vi "Dashboard Main.vi"() -> ()   [LabVIEW 2013]
uses:
  Program Files (x86)/National Instruments/LabVIEW 2013/examples/FRC/Vision/2014 Target Detection/TargetType.ctl
  <vilib>/event_ctls.llb/eventvkey.ctl
  <vilib>/Rock Robotics/WPI/Dashboard/WPI_DashboardLogging Global.vi
  <vilib>/Utility/config.llb/Write Key (String).vi
  <vilib>/Utility/config.llb/Write Key (I32).vi
  <vilib>/Utility/config.llb/NI_LVConfig.lvlib
panel:
  out "Image Message":string="Timeout in Camera Communications"
  in  "Rec Mode":enum32{"Stop", "Record", "Playback"}(radio)
  in  "Dashboard Tab":T1(tab)
  in  "Camera Settings":T2={"Frame Rate"=30, "Compression"=30, "Size"=1} {"Frame Rate" scale=1.0..30.0; "Size" items=["640x480", "320x240", "160x120"]}
  out "MotorSliders R":cluster{"MotorSlide1":dbl, "MotorSlide2":dbl} {"MotorSlide2" scale=-1.0..1.0 scale format="%#_2e"; "MotorSlide1" scale=-1.0..1.0 scale format="%#_2e"}
  out "MotorChart R":cluster{"Numeric":dbl, "Numeric":dbl}(graph)
  out "MotorSliders L":T3 {"MotorSlide4 2" scale=0.0..14.0 scale format="%#_2e"; "MotorSlide2" scale=-1.0..1.0 scale format="%#_2e"; "MotorSlide1" scale=-1.0..1.0 scale format="%#_2e"}
  out "MotorChart L":T4(graph)
  out "JS1 Z":dbl(slide) scale=-1.0..1.0 scale format="%#_2e"
  out "Joystick 1":cluster{"X":dbl, "Y":dbl}[](graph)
  out "JS Buttons 1":T5
  out "JS2 Z":dbl(slide) scale=-1.0..1.0 scale format="%#_2e"
  out "Joystick 2":cluster{"X":dbl, "Y":dbl}[](graph)
  out "JS Buttons 2":T5
  out "Mode":T6(ring)=enum."Auto Disabled"
  out "Camera IP":string
  in  "DB Camera Config":bool
  out "fps":dbl format="%#.1g"
  out "Mbps":dbl format="%#.1g"
  out "Mbps 2":bool
  out "LED 1":bool
  in  "Camera IP":string="10.21.38.11"
  out "Auto To Run":dbl
  in  "Manual Override":bool=TRUE
  out "Halo Sensitivity":dbl=0.75
  out "Ultrasonic":dbl
  in  "Vision Color Controls":T7={"Hue"={110.0, 142.0}, "Sat"={138.0, 255.0}, "Val"={139.0, 198.0}} {"Val" scale=0.0..255.0; "Sat" scale=0.0..255.0; "Hue" scale=0.0..255.0 scale format="%#_3g"}
  out "Distances":T9(array[cluster])
  in  "Test Slider":dbl(slide) scale=0.0..100.0 scale format="%#_3g"
  in  "On/Off":bool caption="Solenoid"
  in  "Test Name":u16(ring) items=["Select the test to run...", "Example Test", "-------------------------------", "List of tests is built in robot code.", "Replace with your own automated tests."]
  in  "Test Tree":string(tree)
  in  "Motor":cluster{"Value":dbl, "Enable":bool} {"Value" scale=-1.0..1.0 scale format="%#_3g"}
  out "Progress":T10 {"Test Progress" scale=0.0..100.0}
  in  "Rev/Fwd":cluster{"Forward":bool, "Reverse":bool}
  in  "Test Ring":u16(ring) items=["Auto", "Fixed indoor", "Fixed outdoor 1", "Fixed outdoor 2", "Fixed fluorescent 1", "Fixed fluorescent 2", "Hold current"]
  in  "Listbox":i32(listbox)
  out "Tree":string(tree)
  out "Camera Image":T11(plugin-control)
  in  "Enable Camera":bool=TRUE
  # "Left"
  # "Front"
  # "Right"
  # "Battery"
  # "Increment with Start,\nDecrement with Back"
  # "Increment with Right D-Pad,\nDecrement with Left D-Pad"
  # "This tab is a great place for autonomous settings and validation.\nCustomize by placing controls and indicators here and name to\nmatch Dashboard Variables on robot."
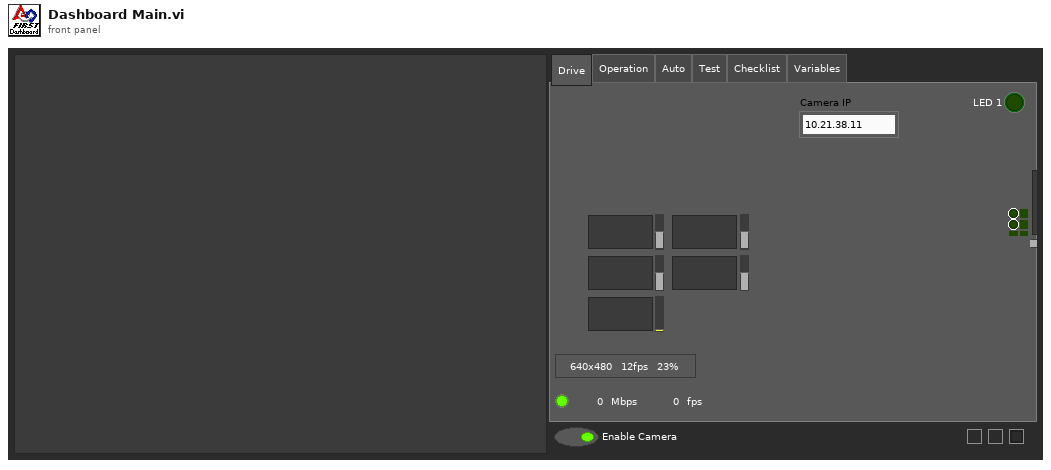
[diagram p1: front panel]
types:
  T1 = enum32{"Drive", "Operation", "Auto", "Test", "Checklist", "Variables"}
  T2 = cluster{"Frame Rate":i32, "Compression":i32, "Size":u16}
  T3 = cluster{"MotorSlide1":dbl, "MotorSlide2":dbl, "MotorSlide4 2":dbl}
  T4 = cluster{"Numeric":dbl, "Numeric":dbl, "Battery":sgl}
  T5 = cluster{bool, bool, bool, bool, bool, bool, bool, bool, bool, bool, bool, bool}
  T6 = enum8{"Tele-Op Disabled", "Tele-Op Enabled", "Auto Disabled", "Auto Enabled", "Test Disabled", "Test Enabled", ""}
  T7 = cluster{"Hue":cluster{dbl, dbl}, "Sat":cluster{dbl, dbl}, "Val":cluster{dbl, dbl}}
  T8 = typedef "TargetType.ctl" = enum16{"Not Hot", "Hot"}
  T9 = cluster{"Distance (ft)":dbl, "Target Center (-1 to 1)":cluster{"X":dbl, "Y":dbl}, "Left":bool, "State":T8}[]
  T10 = cluster{"Test Progress":u8, "Test Progress Text":string}
  T11 = typedef "IMAQ Image.ctl" = refnum<image>
  T12 = typedef "Image Type" = u32
  T13 = cluster{"Digital Inputs":bool[], "Digital Outputs":bool[]}
  T14 = cluster{"Competition mode":bool, "Robot Link":bool, "Autonomous":bool, "Enabled":bool, "E-Stop":bool, "Simulated":bool, "TestMode":bool, "Docked Window":bool}
  T15 = cluster{"Boolean Array[0]":bool, "Boolean Array[1]":bool, "Boolean Array[2]":bool, "Boolean Array[3]":bool, "Boolean Array[4]":bool, "Boolean Array[5]":bool, "Boolean Array[6]":bool, "Boolean Array[7]":bool, "Boolean Array[8]":bool, "Boolean Array[9]":bool, "Boolean Array[10]":bool, "Boolean Array[11]":bool}
  T16 = cluster{cluster{dbl, dbl}, cluster{dbl, dbl}, cluster{dbl, dbl}}
  T17 = typedef "NI_LVConfig.lvlib/Config Data RefNum.ctl" = refnum<k1>
  T18 = typedef "eventvkey.ctl" = enum16{"ASCII", "Enter", "Return", "Shift", "Ctrl", "Alt", "Cmd", "Opt", "Caps", "NumLock", "Clear", "Break", "Up", "Down", "Left", "Right", "Insert", "Delete", "Home", "End", "PageUp", "PageDown", "Escape", "Help", "Pause", "ScrollLock", "F1", "F2", "F3", "F4", "F5", "F6", "F7", "F8", "F9", "F10", "F11", "F12", "F13", "F14", "F15", "F16", "F17", "F18", "F19", "F20", "F21", "F22", "F23", "F24", "Play", "VolumeUp", "VolumeDown", "Mute", "Two Byte Char"}
  T19 = cluster{"Image Size":bool, "Image Type":bool, "Pixel Value":bool, "ROI Information":bool, "Zoom Factor":bool}
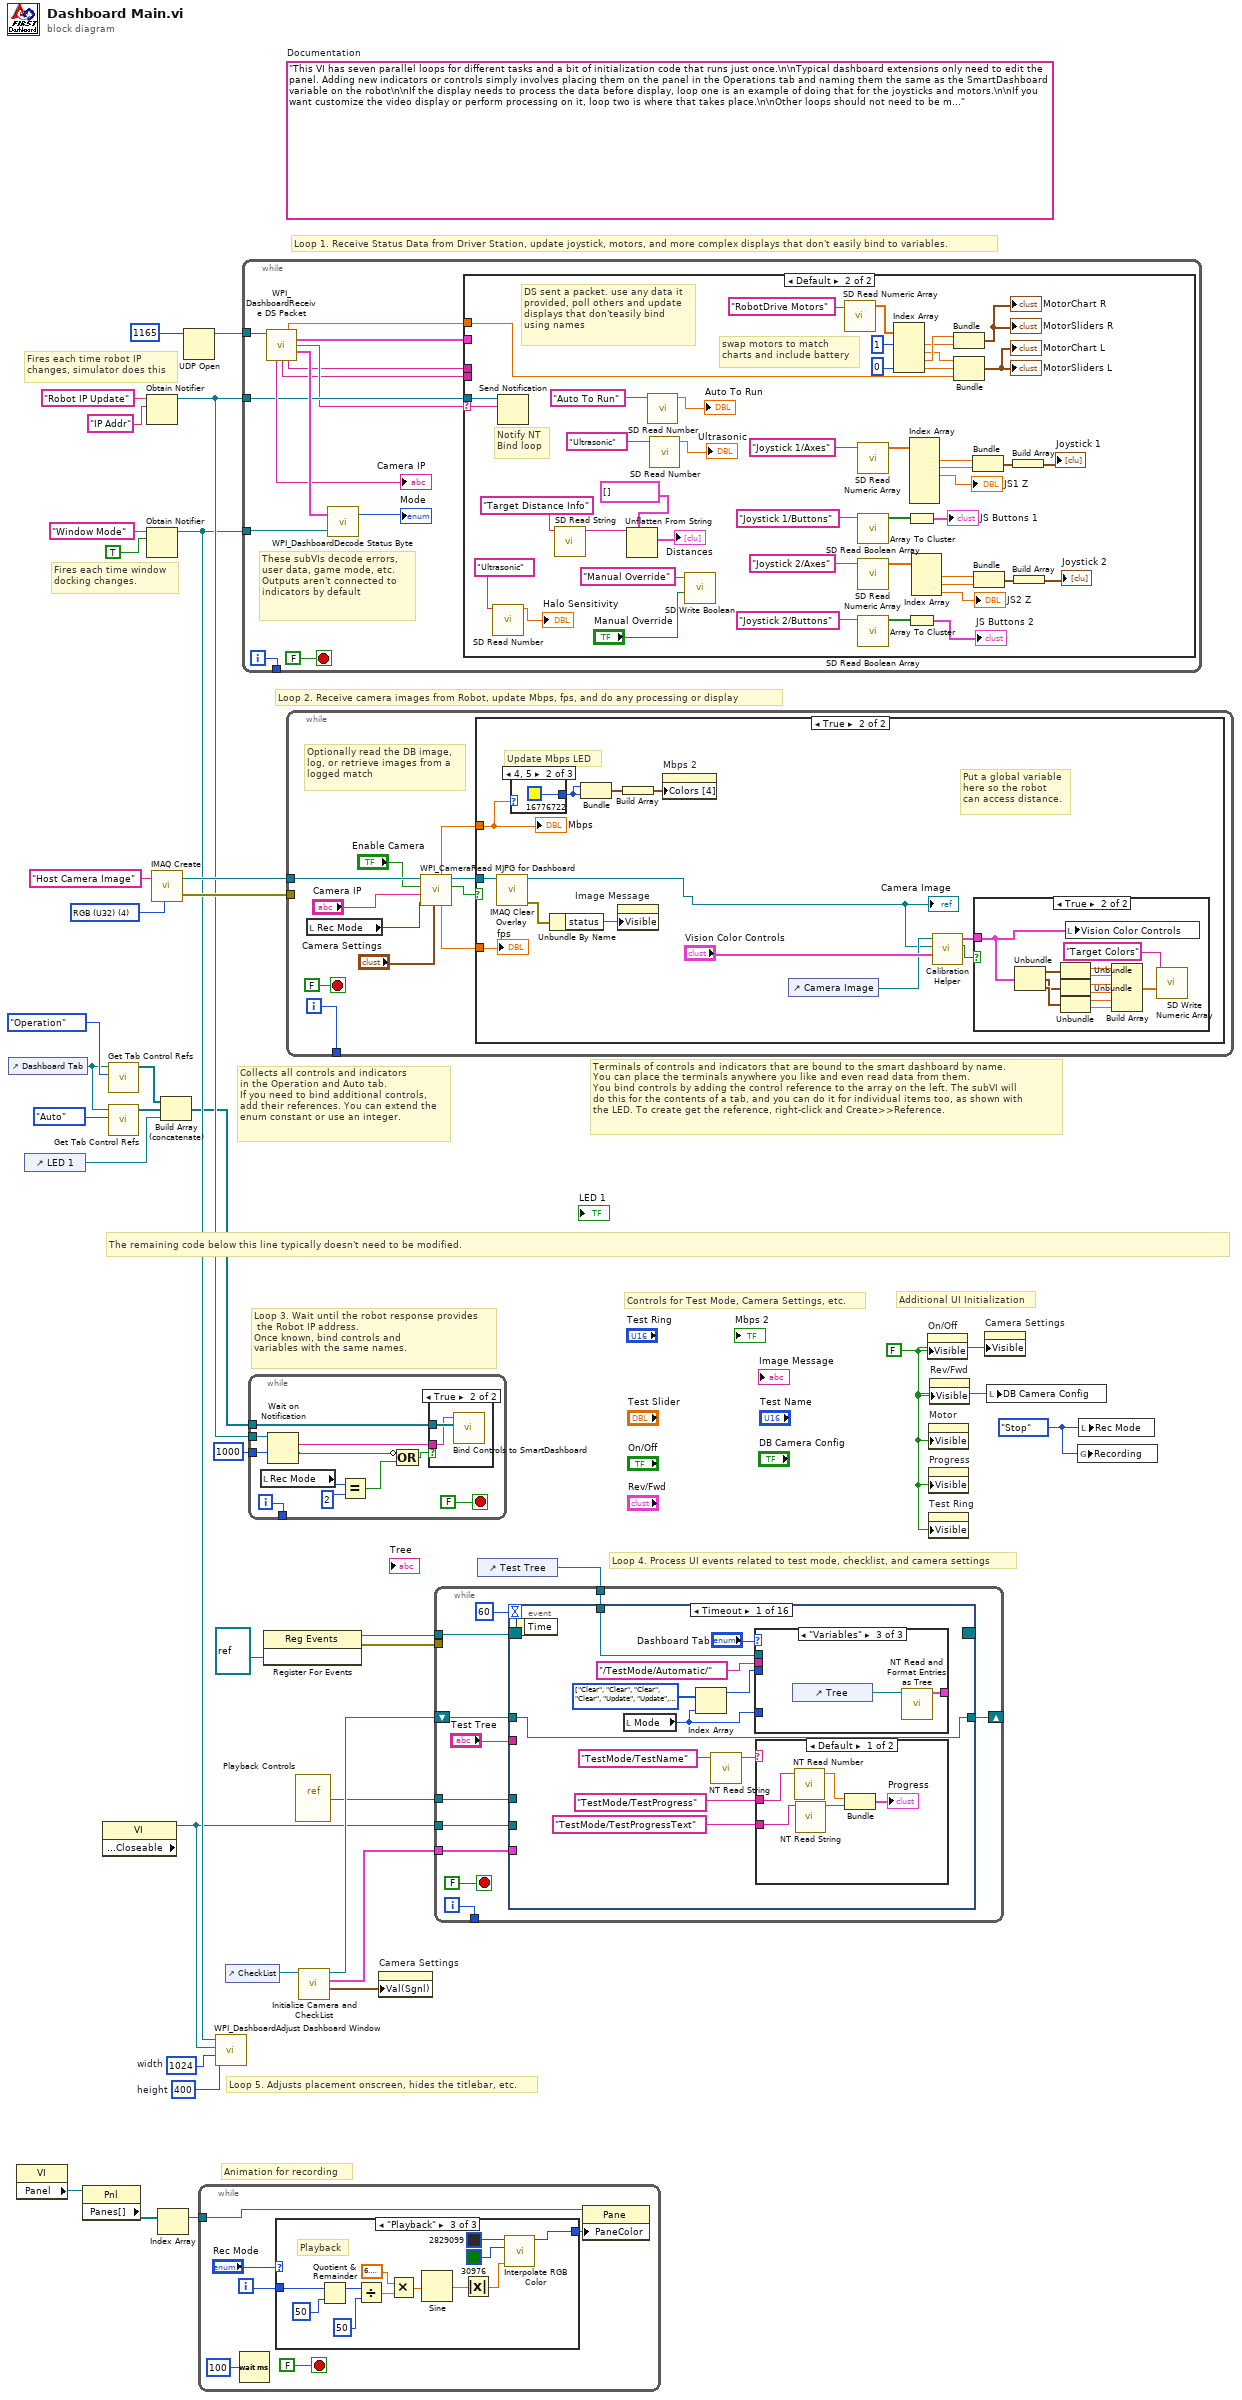
[diagram p0: block diagram]
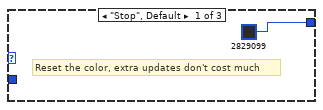
[diagram p2: hidden frame]
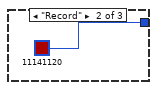
[diagram p3: hidden frame]
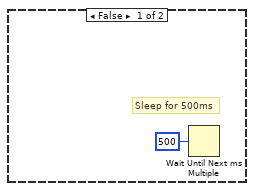
[diagram p5: hidden frame]
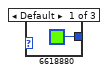
[diagram p7: hidden frame]
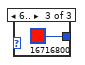
[diagram p8: hidden frame]
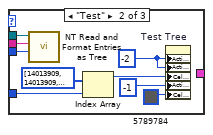
[diagram p10: hidden frame]
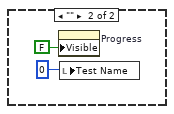
[diagram p11: hidden frame]
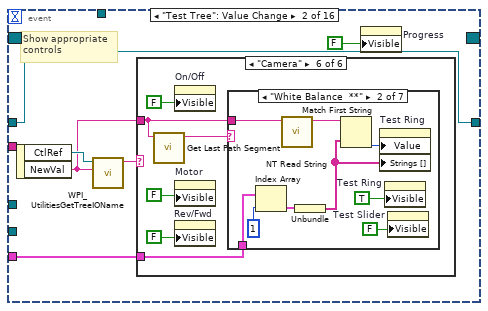
[diagram p12: hidden frame]
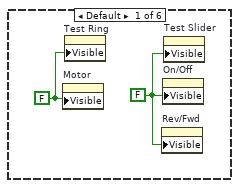
[diagram p13: hidden frame]
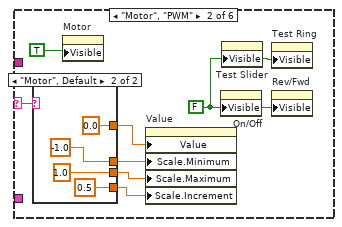
[diagram p14: hidden frame]
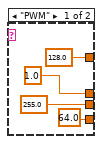
[diagram p15: hidden frame]
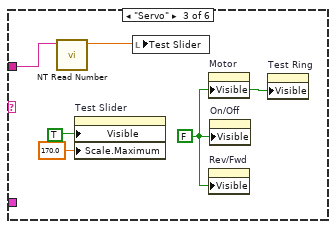
[diagram p16: hidden frame]
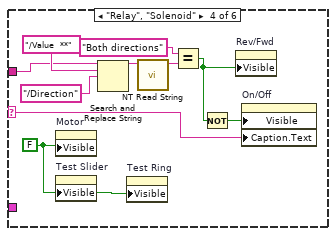
[diagram p17: hidden frame]
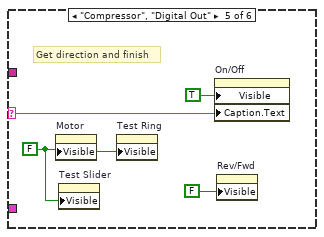
[diagram p18: hidden frame]
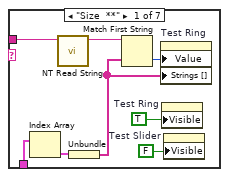
[diagram p19: hidden frame]
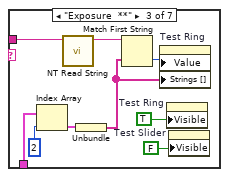
[diagram p20: hidden frame]
diagram:
  w8 = enum32{"Stop", "Record", "Playback"}."Stop" ("Rec Mode")
  w11 = 400  # height
  w12 = 1024  # width
  w25 = FALSE ("Visible")
  (unwired) "This VI has seven parallel loops for different tasks and a bit of initialization code that runs just once.\n\nTypical dashboard extensions only need to edit the panel. Adding new indicators or controls simply involves placing them on the panel in the Operations tab and naming them the same as the SmartDashboard variable on the robot\n\nIf the display needs to process the data before display, loop one is an example of doing that for the joysticks and motors.\n\nIf you want customize the video display or perform processing on it, loop two is where that takes place.\n\nOther loops should not need to be modified. They are pretty standard, and document the task they perform."  # Documentation
  w35 = T12 4 items=["Grayscale (U8)", "Grayscale (I16)", "Grayscale (SGL)", "Complex (CSG)", "RGB (U32)", "HSL (U32)", "RGB (U64)"] ("Image Type")
  # "Controls for Test Mode, Camera Settings, etc."
  # "Additional UI Initialization"
  # "Animation for recording"
  # "Fires each time robot IP\nchanges, simulator does this"
  # "Fires each time window\ndocking changes."
  # "Collects all controls and indicators\nin the Operation and Auto tab.\nIf you need to bind additional controls,\nadd their references. You can extend the\nenum constant or use an integer."
  # "The remaining code below this line typically doesn't need to be modified."
  # "Loop 4. Process UI events related to test mode, checklist, and camera settings"
  # "Terminals of controls and indicators that are bound to the smart dashboard by name.\nYou can place the terminals anywhere you like and even read data from them.\nYou bind controls by adding the control reference to the array on the left. The subVI will\ndo this for the contents of a tab, and you can do it for individual items too, as shown with\nthe LED. To create get the reference, right-click and Create>>Reference."
  # "Loop 3. Wait until the robot response provides\n the Robot IP address.\nOnce known, bind controls and\nvariables with the same names."
  # "Loop 5. Adjusts placement onscreen, hides the titlebar, etc."
  # "Loop 1. Receive Status Data from Driver Station, update joystick, motors, and more complex displays that don't easily bind to variables."
  # "Loop 2. Receive camera images from Robot, update Mbps, fps, and do any processing or display"
  n1 = control-ref of="Dashboard Tab"() -> (w6:refnum<vi>)
  n2 = property class="VI"() -> ("Panel"=w19:refnum<vi>)  [unwired: 2 in, 2 out]
  n3 = control-ref of="LED 1"() -> (w1:refnum<vi>)
  n4 = property class="Pnl"(reference=w19) -> ("Panes[]"=w20:refnum<vi>[])  [unwired: 1 in, 2 out]
  n5 = property class="VI" props=["Front Panel.Closeable"]() -> (reference out=w7:refnum<vi>)  [unwired: 2 in, 2 out]
  n6 = call <vilib>:"Get Tab Control Refs.vi"("Page Index"=T1."Operation" ("Dashboard Tab"), "TabControl in"=w6) -> ("ControlsOnPage"=w4:refnum<vi>[])  [unwired: 9 in]
  n7 = call <vilib>:"Get Tab Control Refs.vi"("Page Index"=T1."Auto" ("Dashboard Tab"), "TabControl in"=w6) -> ("ControlsOnPage"=w5:refnum<vi>[])  [unwired: 9 in]
  n8 = Obtain Notifier(name (unnamed)="Robot IP Update", notification data type="IP Addr" ("name (unnamed)")) -> (notifier out=w29:refnum<notifier>)  [unwired: 2 in, 2 out]
  n9 = Obtain Notifier(name (unnamed)="Window Mode", notification data type=TRUE) -> (notifier out=w10:refnum<notifier>)  [unwired: 2 in, 2 out]
  n10 = call "IMAQ Create"("Image Name"="Host Camera Image", "Image Type"=w35) -> ("New Image"=w33:T11, "error out"=w32:errorcluster)  [unwired: 2 in, 1 out]
  n11 = Index Array(array=w20) -> (element=w18:refnum<vi>)  [unwired: 1 in]
  n12 = Build Array (concatenate)(w4, w5, w1) -> (w3:refnum<vi>[])
  n13 = UDP Open(11:u16 1165 ("port")) -> (port=w36:refnum<k16>)  [unwired: 2 in, 4 out]
  n14 = while {
    tunnel: w18 -> [w39]
    i -> [w42]
    stop <- FALSE stop-if-true
    n15 = Wait (ms)(milliseconds to wait=u32 100) -> ()  [unwired: 1 out]
    n16 = case shown="\"Playback\"" "Rec Mode" {
      tunnel: w42 -> [_ _ w57]
      tunnel: [u32 2829099 ("Base Color") u32 11141120 ("Target Color") w46] -> w38
      frame "Stop", Default {
        # "Reset the color, extra updates don't cost much"
      }
      frame "Record" {
      }
      frame "Playback" {
        # "Playback"
        n17 = Quotient & Remainder(x=w57, y=u32 50 ("milliseconds to wait")) -> (x-y*floor(x/y)=w53:u32)  [unwired: 1 out]
        n18 = Divide(x=w53, y=u32 50 ("milliseconds to wait")) -> (x/y=w50:dbl)
        n19 = Multiply(x=6.283185307179586, y=w50) -> (x*y=w55:dbl)
        n20 = Sine(x=w55) -> (sin(x)=w54:dbl)
        n21 = Absolute Value(x=w54) -> (abs(x)=w47:dbl)
        n22 = call "Interpolate RGB Color.vi"("Proportion"=w47, "Target Color"=u32 30976, "Base Color"=u32 2829099) -> ("Result Color"=w46:u32)  [unwired: 8 in]
      }
    }
    n23 = property class="Pane"(reference=w39, "PaneColor"=w38) -> ()  [unwired: 1 in, 2 out]
  }
  n24 = call <vilib>:"WPI_DashboardAdjust Dashboard Window.vi"("height"=w11, "width"=w12, "reference in"=w7, "Notifier in"=w10) -> ()  [unwired: 8 in]
  n25 = control-ref of="CheckList"() -> (w9:refnum<vi>)
  n26 = while {
    tunnel: w36 -> [w68]
    tunnel: w29 -> [w63]
    tunnel: w10 -> [w67]
    tunnel: [w64] -> _
    i -> [w64]
    stop <- FALSE stop-if-true
    # "These subVIs decode errors, user data, game mode, etc.\nOutputs aren't connected to indicators by default"
    n27 = call <vilib>:"WPI_DashboardReceive DS Packet.vi"("Recv Socket"=w68) -> ("Battery"=w58:sgl, "Driver Station"=w59:T13, "Robot IP Address"=w62:string, "Status"=w69:T14, "Camera IP Address"=→"Camera IP":string, "Low Priority User Data"=w61:string, "High Priority User Data"=w60:string)  [unwired: 1 in, 7 out]
    n28 = call <vilib>:"WPI_DashboardDecode Status Byte.vi"("Window Mode Notifier"=w67, "Status"=w69) -> ("Mode"=→"Mode":T6)  [unwired: 1 out]
    n29 = case shown="Default" w62 {
      selector: w62 -> [_ w94]
      tunnel: w63 -> [_ w95]
      tunnel: w61 -> [_ _]
      tunnel: w60 -> [_ _]
      tunnel: w59 -> [_ _]
      tunnel: w58 -> [_ w93]
      frame "0.0.0.0" {
        # "DS not sending packets, or no robot exists yet.\nDon't poll the variables"
      }
      frame Default {
        # "Notify NT\nBind loop"
        # "DS sent a packet. use any data it\nprovided, poll others and update\ndisplays that don'teasily bind\nusing names"
        # "swap motors to match\ncharts and include battery"
        n30 = call <vilib>:"SD Read Number.vi"("Name"="Ultrasonic") -> ("Numeric"=→"Halo Sensitivity":dbl)  [unwired: 8 in, 2 out]
        n31 = Send Notification(notification=w94, notifier=w95) -> ()  [unwired: 1 in, 2 out]
        n32 = call <vilib>:"SD Read String.vi"("Name"="Target Distance Info") -> ("String"=w80:string)  [unwired: 8 in, 2 out]
        n33 = Unflatten From String(type=T9 [] ("Distances"), binary string=w80) -> (value=→"Distances":T9)  [unwired: 3 in, 2 out]
        n34 = call <vilib>:"SD Read Number.vi"("Name"="Auto To Run") -> ("Numeric"=→"Auto To Run":dbl)  [unwired: 8 in, 2 out]
        n35 = call <vilib>:"SD Read Number.vi"("Name"="Ultrasonic") -> ("Numeric"=→"Ultrasonic":dbl)  [unwired: 8 in, 2 out]
        n36 = call <vilib>:"SD Write Boolean.vi"("Boolean"="Manual Override", "Name"="Manual Override") -> ()  [unwired: 8 in, 2 out]
        n37 = call <vilib>:"SD Read Numeric Array.vi"("Name"="RobotDrive Motors") -> ("Numeric Array"=w92:dbl[])  [unwired: 8 in, 2 out]
        n38 = call <vilib>:"SD Read Numeric Array.vi"("Name"="Joystick 1/Axes") -> ("Numeric Array"=w110:dbl[])  [unwired: 8 in, 2 out]
        n39 = call <vilib>:"SD Read Boolean Array.vi"("Name"="Joystick 1/Buttons") -> ("Boolean Array"=w112:bool[])  [unwired: 8 in, 2 out]
        n40 = call <vilib>:"SD Read Numeric Array.vi"("Name"="Joystick 2/Axes") -> ("Numeric Array"=w105:dbl[])  [unwired: 8 in, 2 out]
        n41 = call <vilib>:"SD Read Boolean Array.vi"("Name"="Joystick 2/Buttons") -> ("Boolean Array"=w104:bool[])  [unwired: 8 in, 2 out]
        n42 = Index Array(array=w92, index #1=1, index #4=0) -> (element #1=w88:dbl, element #2=w87:dbl, element #3=w89:dbl, element #4=w84:dbl)  [unwired: 2 in]
        n43 = Array To Cluster(array=w112) -> (cluster=→"JS Buttons 1":T15)
        n44 = Array To Cluster(array=w104) -> (cluster=→"JS Buttons 2":T15)
        n45 = Index Array(array=w110) -> (element #1=w108:dbl, element #2=w79:dbl, element #3=→"JS1 Z":dbl)  [unwired: 6 in, 3 out]
        n46 = Index Array(array=w105) -> (element #1=w100:dbl, element #2=w99:dbl, element #3=→"JS2 Z":dbl)  [unwired: 3 in]
        n47 = Bundle("Numeric"=w89, "Numeric"=w88) -> (→"MotorChart R" →"MotorSliders R":cluster{"Numeric":dbl, "Numeric":dbl})  [unwired: 1 in]
        n48 = Bundle("Numeric"=w87, "Numeric"=w84, "Battery"=w93) -> (→"MotorChart L" →"MotorSliders L":T4)  [unwired: 1 in]
        n49 = Bundle("Numeric"=w108, "Numeric"=w79) -> (w107:cluster{"Numeric":dbl, "Numeric":dbl})  [unwired: 1 in]
        n50 = Bundle("Numeric"=w100, "Numeric"=w99) -> (w101:cluster{"Numeric":dbl, "Numeric":dbl})  [unwired: 1 in]
        n51 = Build Array(w107) -> (→"Joystick 1":cluster{"Numeric":dbl, "Numeric":dbl}[])
        n52 = Build Array(w101) -> (→"Joystick 2":cluster{"Numeric":dbl, "Numeric":dbl}[])
      }
    }
  }
  n53 = while {
    tunnel: w3 -> [w126]
    tunnel: w29 -> [w124]
    tunnel: [w122] -> _
    tunnel: u32 1000 ("milliseconds to wait") -> [w121]
    i -> [w122]
    stop <- FALSE stop-if-true
    n54 = local read "Rec Mode"() -> (w117:enum32{"Stop", "Record", "Playback"})
    n55 = Wait on Notification(notifier=w124, timeout in ms (-1)=w121) -> (notification=w123:string, timed out?=w119:bool)  [unwired: 2 in, 2 out]
    n56 = Equal?(x=w117, y=u16 2 ("Rec Mode")) -> (x = y?=w118:bool)
    n57 = Compound Arithmetic op=OR(invert w119, w118) -> (w120:bool)
    n58 = case shown="True" w120 {
      tunnel: w126 -> [_ w128]
      tunnel: w123 -> [_ w127]
      frame False {
      }
      frame True {
        n59 = call <vilib>:"Bind Controls to SmartDashboard.vi"("Bound Control Refs"=w128, "Server IP Address"=w127) -> ()  [unwired: 10 in]
      }
    }
  }
  n60 = register-events(refnum<vi> refnum) -> (reference out=w16:refnum<event-registration>, error out=w15:errorcluster)  [unwired: 2 in]
  n61 = while {
    tunnel: w33 -> [w137]
    tunnel: w32 -> [_]
    tunnel: [w138] -> _
    i -> [w138]
    stop <- FALSE stop-if-true
    # "Optionally read the DB image,\nlog, or retrieve images from a\nlogged match"
    n62 = local read "Rec Mode"() -> (w130:enum32{"Stop", "Record", "Playback"})
    n63 = call <vilib>:"WPI_CameraRead MJPG for Dashboard.vi"("Camera Settings"="Camera Settings", "Rec Mode"=w130, "Camera IP"="Camera IP", "Enable"="Enable Camera", "Refnum in"=w137) -> ("Active"=w134:bool, "Refnum out"=w136:T11, "FPS"=w133:dbl, "Bandwidth (Mbps)"=w132:dbl)  [unwired: 3 in]
    n64 = case shown="True" w134 {
      tunnel: w136 -> [_ w148]
      tunnel: w132 -> [_ w147]
      tunnel: w133 -> [_ w146]
      frame False {
        # "Sleep for 500ms"
        n65 = Wait Until Next ms Multiple(millisecond multiple=u32 500) -> ()  [unwired: 1 out]
      }
      frame True {
        # "Put a global variable\nhere so the robot\ncan access distance."
        # "Update Mbps LED"
        n66 = call "IMAQ Clear Overlay"("Image"=w148) -> ("error out"=w152:errorcluster, "Image Out"=w141:T11)  [unwired: 2 in, 7 out]
        "Camera Image" <- w141
        n67 = case shown="4, 5" w147 {
          tunnel: [u32 6618880 ("Color Box") u32 16776722 ("Color Box") u32 16716800 ("Color Box")] -> w149
          frame Default {
          }
          frame 4, 5 {
          }
          frame 6.. {
          }
        }
        n68 = Unbundle By Name(w152) -> ("status"=w153:bool)
        n69 = Bundle("Color Box"=w149, "Color Box"=w149) -> (w151:cluster{"Color Box":u32, "Color Box":u32})  [unwired: 1 out]
        n70 = property on="Image Message" class="Str"("Visible"=w153) -> ()  [unwired: 2 in, 2 out]
        n71 = Build Array(w151) -> (w150:cluster{"Color Box":u32, "Color Box":u32}[])
        n72 = property on="Mbps 2" class="Bool (strict)"("Colors [4]"=w150) -> ()  [unwired: 2 in, 2 out]
        n73 = control-ref of="Camera Image"() -> (w143:refnum<vi>)
        n74 = call "Calibration Helper.vi"("Color Components"="Vision Color Controls", "Image"=w141, "Image Ctl Refnum"=w143) -> ("Changed"=w142:bool, "output color"=w144:T16)  [unwired: 7 in]
        n75 = case shown="True" w142 {
          tunnel: w144 -> [_ w165]
          frame False {
          }
          frame True {
            n76 = Unbundle(w165) -> (w164:cluster{dbl, dbl}, w159:cluster{dbl, dbl}, w163:cluster{dbl, dbl})
            n77 = Unbundle(w164) -> (w162:dbl, w161:dbl)
            n78 = Unbundle(w159) -> (w160:dbl, w158:dbl)
            n79 = Unbundle(w163) -> (w157:dbl, w156:dbl)
            n80 = local write "Vision Color Controls"(w165) -> ()
            n81 = Build Array(w162, w161, w160, w158, w157, w156) -> (w155:dbl[])
            n82 = call <vilib>:"SD Write Numeric Array.vi"("Numeric Array"=w155, "Name"="Target Colors") -> ()  [unwired: 8 in, 2 out]
          }
        }
        "Mbps" <- w147
        "fps" <- w146
      }
    }
  }
  n83 = vi-ref "Playback Controls.vi"() -> (w17:refnum<vi>)
  n84 = call "Initialize Camera and CheckList.vi"("ListBox in"=w9) -> ("Cluster"=w23:cluster{"value":i32, "value":i32, "index":i32}, "Array"=w24:cluster{string[]}[], "File Refnum"=w22:T17)  [unwired: 8 in]
  n85 = property on="Camera Settings" class="Clust (strict)"("Val(Sgnl)"=w23) -> ()  [unwired: 2 in, 2 out]
  n86 = control-ref of="Test Tree"() -> (w21:refnum<vi>)
  n87 = while {
    tunnel: w24 -> [w176]
    shift-right: [w175] -> _
    shift-left: w22 -> [w174]
    tunnel: [w173] -> _
    tunnel: w21 -> [w172]
    tunnel: w17 -> [w171]
    tunnel: w16 -> [w170]
    tunnel: w15 -> [_]
    tunnel: w7 -> [w169]
    i -> [w173]
    stop <- FALSE stop-if-true
    n88 = event shown="[0] Timeout" {
      selector: w170 -> [_ _ _ _ _ _ _ _ _ _ _ _ _ _ _ _]
      dyn-events: [_ _ _ _ _ _ _ _ _ _ _ _ _ w414 _ _] -> _
      timeout: u32 60 ("milliseconds to wait") -> [_ _ _ _ _ _ _ _ _ _ _ _ _ _ _ _]
      tunnel: w172 -> [w186 _ _ _ _ _ _ _ _ _ _ _ _ _ _ _]
      tunnel: "Test Tree" -> [_ _ _ _ _ _ _ _ w383 w391 w393 w397 w405 _ _ _]
      tunnel: w176 -> [_ w210 _ _ _ _ w347 w377 _ _ _ _ _ _ _ _]
      tunnel: [w180 w209 w308 w313 w321 w333 w346 w370 w382 w389 w392 w396 w404 w416 w430 w431] -> w175
      tunnel: w174 -> [w180 w209 w308 w313 w321 w333 w345 w370 w382 w389 w392 w396 w404 w416 w430 w431]
      tunnel: w171 -> [_ _ _ _ _ _ _ _ _ _ _ _ _ w417 _ w434]
      tunnel: w169 -> [_ _ _ _ _ _ _ _ _ _ _ _ _ w412 _ _]
      event Timeout {
        w185 = enum16{"Update", "Clear"}[] [enum."Clear", enum."Clear", enum."Clear", enum."Clear", enum."Update", enum."Update", enum."Clear"] items=["Update", "Clear"]
        n89 = event-data() -> ()  [unwired: 1 in, 1 out]
        n90 = local read "Mode"() -> (w183:T6)
        n91 = Index Array(array=w185, index=w183) -> (element=w184:enum16{"Update", "Clear"})
        n92 = call <vilib>:"NT Read String.vi"("Name"="TestMode/TestName") -> ("String"=w189:string)  [unwired: 9 in, 1 out]
        n93 = case shown="\"Variables\"" "Dashboard Tab" {
          tunnel: w186 -> [_ w199 _]
          tunnel: "/TestMode/Automatic/" ("Name Pattern") -> [_ w198 _]
          tunnel: w184 -> [_ w197 _]
          tunnel: w183 -> [_ w195 _]
          tunnel: [_ _ w201] -> _
          frame "Operation", Default {
          }
          frame "Test" {
            w194 = -2 ("Active Item:Row Number")
            n94 = call <vilib>:"NT Read and Format Entries as Tree.vi"("Operation"=w197, "Name Pattern"=w198, "Tree Refnum"=w199) -> ()  [unwired: 7 in, 2 out]
            n95 = Index Array(array=u32[] [14013909, 14013909, 14013909, 14013909, 14013909, 16777215, 14013909], index=w195) -> (element=w193:u32)
            n96 = property on="Test Tree" class="Tree (strict)"("Active Item Row Number"=w194, "ActiveColNum"=w194, "CellBG"=w193, "Active Item Row Number"=-1 ("Active Item:Row Number"), "CellBG"=u32 5789784 ("Color Box")) -> ()  [unwired: 2 in, 2 out]
          }
          frame "Variables" {
            n97 = control-ref of="Tree"() -> (w200:refnum<vi>)
            n98 = call <vilib>:"NT Read and Format Entries as Tree.vi"("Tree Refnum"=w200) -> ("Formatted Strings"=w201:cluster{"Name":string, "Value":string}[])  [unwired: 9 in, 1 out]
          }
        }
        n99 = case shown="Default" w189 {
          tunnel: "TestMode/TestProgress" ("Name") -> [w203 _]
          tunnel: "TestMode/TestProgressText" ("Name") -> [w202 _]
          frame Default {
            n100 = call <vilib>:"NT Read Number.vi"("Name"=w203) -> ("Numeric"=w204:dbl)  [unwired: 9 in, 1 out]
            n101 = call <vilib>:"NT Read String.vi"("Name"=w202) -> ("String"=w205:string)  [unwired: 9 in, 1 out]
            n102 = Bundle("Numeric"=w204, "String"=w205) -> (→"Progress":cluster{"Numeric":dbl, "String":string})  [unwired: 1 in]
          }
          frame "" {
            n103 = property on="Progress" class="Clust (strict)"("Visible"=FALSE) -> ()  [unwired: 2 in, 2 out]
            n104 = local write "Test Name"(u16 0) -> ()
          }
        }
      }
      event "Test Tree": Value Change {
        # "Show appropriate\ncontrols"
        n105 = event-data() -> ("CtlRef"=w213:refnum<vi>, "NewVal"=w211:string)  [unwired: 1 in]
        n106 = call <vilib>:"WPI_UtilitiesGetTreeIOName.vi"("NewVal"=w211, "TreeControl in"=w213) -> ("I/O Name"=w214:string)  [unwired: 9 in]
        n107 = case shown="\"Camera\"" w214 {
          selector: w214 -> [_ w221 _ w239 w248 _]
          tunnel: w211 -> [_ _ w236 w238 _ w255]
          tunnel: w210 -> [_ _ _ _ _ w254]
          frame Default {
            w216 = FALSE ("Visible")
            w215 = FALSE ("Visible")
            n108 = property on="Motor" class="Clust (strict)"("Visible"=w215) -> ()  [unwired: 2 in, 2 out]
            n109 = property on="Test Ring" class="Ring (strict)"("Visible"=w215) -> ()  [unwired: 2 in, 2 out]
            n110 = property on="Rev/Fwd" class="Clust (strict)"("Visible"=w216) -> ()  [unwired: 2 in, 2 out]
            n111 = property on="On/Off" class="Bool (strict)"("Visible"=w216) -> ()  [unwired: 2 in, 2 out]
            n112 = property on="Test Slider" class="Slide (strict)"("Visible"=w216) -> ()  [unwired: 2 in, 2 out]
          }
          frame "Motor", "PWM" {
            w222 = FALSE ("Visible")
            n113 = case shown="\"Motor\", Default" w221 {
              tunnel: [1.0 ("Value") -1.0 ("Value")] -> w220
              tunnel: [255.0 ("Value") 1.0 ("Value")] -> w219
              tunnel: [128.0 ("Value") 0.0 ("Value")] -> w218
              tunnel: [64.0 ("Value") 0.5 ("Value")] -> w217
              frame "PWM" {
              }
              frame "Motor", Default {
              }
            }
            n114 = property on="Motor" class="Clust (strict)"("Visible"=TRUE) -> ()  [unwired: 2 in, 2 out]
            n115 = property on="Value" class="Slide (strict)"("Value"=w218, "Scale.Minimum"=w220, "Scale.Maximum"=w219, "Scale.Increment"=w217) -> ()  [unwired: 2 in, 2 out]
            n116 = property on="On/Off" class="Bool (strict)"("Visible"=w222) -> ()  [unwired: 2 in, 2 out]
            n117 = property on="Test Slider" class="Slide (strict)"("Visible"=w222) -> ()  [unwired: 2 in, 2 out]
            n118 = property on="Test Ring" class="Ring (strict)"("Visible"=w222) -> ()  [unwired: 2 in, 2 out]
            n119 = property on="Rev/Fwd" class="Clust (strict)"("Visible"=w222) -> ()  [unwired: 2 in, 2 out]
          }
          frame "Servo" {
            w234 = FALSE ("Visible")
            n120 = call <vilib>:"NT Read Number.vi"("Name"=w236) -> ("Numeric"=w235:dbl)  [unwired: 9 in, 1 out]
            n121 = property on="Test Slider" class="Slide (strict)"("Visible"=TRUE, "Scale.Maximum"=170.0 ("Scale.Range:Maximum")) -> ()  [unwired: 2 in, 2 out]
            n122 = local write "Test Slider"(w235) -> ()
            n123 = property on="Motor" class="Clust (strict)"("Visible"=w234) -> ()  [unwired: 2 in, 2 out]
            n124 = property on="Rev/Fwd" class="Clust (strict)"("Visible"=w234) -> ()  [unwired: 2 in, 2 out]
            n125 = property on="On/Off" class="Bool (strict)"("Visible"=w234) -> ()  [unwired: 2 in, 2 out]
            n126 = property on="Test Ring" class="Ring (strict)"("Visible"=w234) -> ()  [unwired: 2 in, 2 out]
          }
          frame "Relay", "Solenoid" {
            w237 = FALSE ("Visible")
            n127 = property on="Motor" class="Clust (strict)"("Visible"=w237) -> ()  [unwired: 2 in, 2 out]
            n128 = property on="Test Slider" class="Slide (strict)"("Visible"=w237) -> ()  [unwired: 2 in, 2 out]
            n129 = Search and Replace String(input string=w238, search string="/Value  **", replace string="/Direction") -> (result string=w244:string)  [unwired: 5 in, 3 out]
            n130 = property on="Test Ring" class="Ring (strict)"("Visible"=w237) -> ()  [unwired: 2 in, 2 out]
            n131 = call <vilib>:"NT Read String.vi"("Name"=w244) -> ("String"=w242:string)  [unwired: 9 in, 1 out]
            n132 = Equal?(x="Both directions", y=w242) -> (x = y?=w240:bool)
            n133 = Not(x=w240) -> (.not. x?=w241:bool)
            n134 = property on="Rev/Fwd" class="Clust (strict)"("Visible"=w240) -> ()  [unwired: 2 in, 2 out]
            n135 = property on="On/Off" class="Bool (strict)"("Visible"=w241, "Caption.Text"=w239) -> ()  [unwired: 2 in, 2 out]
          }
          frame "Compressor", "Digital Out" {
            w247 = FALSE ("Visible")
            # "Get direction and finish"
            n136 = property on="Motor" class="Clust (strict)"("Visible"=w247) -> ()  [unwired: 2 in, 2 out]
            n137 = property on="Test Slider" class="Slide (strict)"("Visible"=w247) -> ()  [unwired: 2 in, 2 out]
            n138 = property on="Test Ring" class="Ring (strict)"("Visible"=w247) -> ()  [unwired: 2 in, 2 out]
            n139 = property on="On/Off" class="Bool (strict)"("Visible"=TRUE, "Caption.Text"=w248) -> ()  [unwired: 2 in, 2 out]
            n140 = property on="Rev/Fwd" class="Clust (strict)"("Visible"=FALSE) -> ()  [unwired: 2 in, 2 out]
          }
          frame "Camera" {
            n141 = call <vilib>:"Get Last Path Segment.vi"("String in"=w255) -> ("String out"=w256:string)  [unwired: 10 in]
            n142 = property on="On/Off" class="Bool (strict)"("Visible"=FALSE) -> ()  [unwired: 2 in, 2 out]
            n143 = property on="Motor" class="Clust (strict)"("Visible"=FALSE) -> ()  [unwired: 2 in, 2 out]
            n144 = property on="Rev/Fwd" class="Clust (strict)"("Visible"=FALSE) -> ()  [unwired: 2 in, 2 out]
            n145 = case shown="\"White Balance  **\"" w256 {
              tunnel: w255 -> [w262 w271 w280 w289 w298 _ w304]
              tunnel: w254 -> [w260 w268 w277 w286 w295 _ _]
              frame "Size  **" {
                n146 = Index Array(array=w260) -> (element=w259:cluster{string[]})  [unwired: 1 in]
                n147 = call <vilib>:"NT Read String.vi"("Name"=w262) -> ("String"=w261:string)  [unwired: 9 in, 1 out]
                n148 = Unbundle(w259) -> (w257:string[])
                n149 = Match First String(2:w257, 3:w261) -> (0:w258:i32)  [unwired: 1 out]
                n150 = property on="Test Ring" class="Ring (strict)"("Value"=w258, "Strings []"=w257) -> ()  [unwired: 2 in, 2 out]
                n151 = property on="Test Ring" class="Ring (strict)"("Visible"=TRUE) -> ()  [unwired: 2 in, 2 out]
                n152 = property on="Test Slider" class="Slide (strict)"("Visible"=FALSE) -> ()  [unwired: 2 in, 2 out]
              }
              frame "White Balance  **" {
                n153 = Index Array(array=w268, index=1) -> (element=w269:cluster{string[]})
                n154 = call <vilib>:"NT Read String.vi"("Name"=w271) -> ("String"=w270:string)  [unwired: 9 in, 1 out]
                n155 = Unbundle(w269) -> (w266:string[])
                n156 = Match First String(2:w266, 3:w270) -> (0:w265:i32)  [unwired: 1 out]
                n157 = property on="Test Ring" class="Ring (strict)"("Value"=w265, "Strings []"=w266) -> ()  [unwired: 2 in, 2 out]
                n158 = property on="Test Ring" class="Ring (strict)"("Visible"=TRUE) -> ()  [unwired: 2 in, 2 out]
                n159 = property on="Test Slider" class="Slide (strict)"("Visible"=FALSE) -> ()  [unwired: 2 in, 2 out]
              }
              frame "Exposure  **" {
                n160 = Index Array(array=w277, index=2) -> (element=w278:cluster{string[]})
                n161 = call <vilib>:"NT Read String.vi"("Name"=w280) -> ("String"=w279:string)  [unwired: 9 in, 1 out]
                n162 = Unbundle(w278) -> (w274:string[])
                n163 = Match First String(2:w274, 3:w279) -> (0:w275:i32)  [unwired: 1 out]
                n164 = property on="Test Ring" class="Ring (strict)"("Value"=w275, "Strings []"=w274) -> ()  [unwired: 2 in, 2 out]
                n165 = property on="Test Ring" class="Ring (strict)"("Visible"=TRUE) -> ()  [unwired: 2 in, 2 out]
                n166 = property on="Test Slider" class="Slide (strict)"("Visible"=FALSE) -> ()  [unwired: 2 in, 2 out]
              }
              frame "Exposure Priority  **" {
                n167 = Index Array(array=w286, index=3) -> (element=w287:cluster{string[]})
                n168 = call <vilib>:"NT Read String.vi"("Name"=w289) -> ("String"=w288:string)  [unwired: 9 in, 1 out]
                n169 = Unbundle(w287) -> (w283:string[])
                n170 = Match First String(2:w283, 3:w288) -> (0:w284:i32)  [unwired: 1 out]
                n171 = property on="Test Ring" class="Ring (strict)"("Value"=w284, "Strings []"=w283) -> ()  [unwired: 2 in, 2 out]
                n172 = property on="Test Ring" class="Ring (strict)"("Visible"=TRUE) -> ()  [unwired: 2 in, 2 out]
                n173 = property on="Test Slider" class="Slide (strict)"("Visible"=FALSE) -> ()  [unwired: 2 in, 2 out]
              }
              frame "Color Enable  **" {
                n174 = Index Array(array=w295, index=4) -> (element=w296:cluster{string[]})
                n175 = call <vilib>:"NT Read String.vi"("Name"=w298) -> ("String"=w297:string)  [unwired: 9 in, 1 out]
                n176 = Unbundle(w296) -> (w292:string[])
                n177 = Match First String(2:w292, 3:w297) -> (0:w293:i32)  [unwired: 1 out]
                n178 = property on="Test Ring" class="Ring (strict)"("Value"=w293, "Strings []"=w292) -> ()  [unwired: 2 in, 2 out]
                n179 = property on="Test Ring" class="Ring (strict)"("Visible"=TRUE) -> ()  [unwired: 2 in, 2 out]
                n180 = property on="Test Slider" class="Slide (strict)"("Visible"=FALSE) -> ()  [unwired: 2 in, 2 out]
              }
              frame Default {
                n181 = property on="Test Ring" class="Ring (strict)"("Visible"=FALSE) -> ()  [unwired: 2 in, 2 out]
                n182 = property on="Test Slider" class="Slide (strict)"("Visible"=FALSE) -> ()  [unwired: 2 in, 2 out]
              }
              frame "Brightness  **", "Color Level  **", "Compression  **", "FPS  **", "Sharpness  **" {
                n183 = call <vilib>:"NT Read Number.vi"("Name"=w304) -> ("Numeric"=w303:dbl)  [unwired: 9 in, 1 out]
                n184 = local write "Test Slider"(w303) -> ()
                n185 = property on="Test Slider" class="Slide (strict)"("Visible"=TRUE, "Scale.Maximum"=100.0 ("Scale.Range:Maximum")) -> ()  [unwired: 2 in, 2 out]
                n186 = property on="Test Ring" class="Ring (strict)"("Visible"=FALSE) -> ()  [unwired: 2 in, 2 out]
              }
            }
          }
        }
        n187 = property on="Progress" class="Clust (strict)"("Visible"=FALSE) -> ()  [unwired: 2 in, 2 out]
      }
      event "Test Name": Mouse Enter {
        # "Populate the ring with the list of tests"
        n188 = event-data() -> ()  [unwired: 1 in, 1 out]
        n189 = call <vilib>:"NT Read String Array.vi"("Name"="TestMode/TestList") -> ("String Array"=w312:string[])  [unwired: 9 in, 1 out]
        n190 = Build Array (concatenate)("Select the test to run...", w312) -> (w311:string[])
        n191 = property on="Test Name" class="Ring (strict)"("Strings []"=w311) -> ()  [unwired: 2 in, 2 out]
      }
      event "Test Name": Value Change {
        w314 = FALSE ("Visible")
        # "Tell the robot the test name to run"
        n192 = event-data() -> ("NewVal"=w318:u16)  [unwired: 1 in]
        n193 = property on="Test Name" class="Ring (strict)"() -> ("Strings []"=w319:string[])  [unwired: 2 in, 2 out]
        n194 = local write "Progress"(T10 {"Test Progress"=0, "Test Progress Text"=""} ("Progress")) -> ()
        n195 = Index Array(array=w319, index=w318) -> (element=w317:string)
        n196 = call <vilib>:"NT Write String.vi"("String"=w317, "Name"="TestMode/TestName") -> ()  [unwired: 9 in, 1 out]
        n197 = property on="Progress" class="Clust (strict)"("Visible"=TRUE) -> ()  [unwired: 2 in, 2 out]
        n198 = property on="Motor" class="Clust (strict)"("Visible"=w314) -> ()  [unwired: 2 in, 2 out]
        n199 = property on="Test Slider" class="Slide (strict)"("Visible"=w314) -> ()  [unwired: 2 in, 2 out]
        n200 = property on="On/Off" class="Bool (strict)"("Visible"=w314) -> ()  [unwired: 2 in, 2 out]
        n201 = property on="Rev/Fwd" class="Clust (strict)"("Visible"=w314) -> ()  [unwired: 2 in, 2 out]
        n202 = property on="Test Ring" class="Ring (strict)"("Visible"=w314) -> ()  [unwired: 2 in, 2 out]
      }
      event "Listbox": Double Click {
        n203 = event-data() -> ("PlatMods.Shift"=w322:bool, "Row"=w324:i32)  [unwired: 1 in]
        n204 = case shown="True" w322 {
          tunnel: w324 -> [w328 _]
          tunnel: 1 -> [w327 _]
          frame False {
            n205 = property on="Listbox" class="LstBox (strict)"() -> ("Item Symbols"=w326:i32[])  [unwired: 2 in, 2 out]
            n206 = Replace Array Subset(array=w326, new element=w327, index=w328) -> (w325:i32[])
            n207 = property on="Listbox" class="LstBox (strict)"("Item Symbols"=w325) -> ()  [unwired: 2 in, 2 out]
          }
          frame True {
            w329 = 0 ("Top Row")
            n208 = property on="Listbox" class="LstBox (strict)"() -> ("Number of Rows"=w331:u32)  [unwired: 2 in, 2 out]
            n209 = Initialize Array(0, w331) -> (w330:i32[])
            n210 = property on="Listbox" class="LstBox (strict)"("Top Row"=w329, "Value"=w329, "Item Symbols"=w330) -> ()  [unwired: 2 in, 2 out]
          }
        }
      }
      event "Listbox": Key Down {
        n211 = event-data() -> ("VKey"=w335:T18)  [unwired: 1 in]
        n212 = case shown="\"Left\", \"Right\"" w335 {
          selector: w335 -> [w340 _]
          tunnel: eventvkey."Left" ("VKey") -> [w338 _]
          frame "Left", "Right" {
            n213 = Equal?(x=w338, y=w340) -> (x = y?=w339:bool)
            n214 = Select(t=0, s=w339, f=1) -> (s? t:f=w341:i32)
            n215 = property on="Listbox" class="LstBox (strict)"() -> ("Item Symbols"=w344:i32[])  [unwired: 2 in, 2 out]
            n216 = Replace Array Subset(array=w344, new element=w341, index="Listbox") -> (w343:i32[])
            n217 = property on="Listbox" class="LstBox (strict)"("Item Symbols"=w343) -> ()  [unwired: 2 in, 2 out]
          }
          frame Default {
          }
        }
      }
      event "DB Camera Config": Value Change {
        n218 = event-data() -> ("NewVal"=w348:bool)  [unwired: 1 in]
        n219 = case shown="False" w348 {
          tunnel: w347 -> [w357 _]
          tunnel: [w350 w368] -> w346
          tunnel: w345 -> [w349 w368]
          frame False {
            w364 = "Camera"
            w367 = FALSE ("Visible")
            n220 = local read "Camera Settings"() -> (w356:T2)
            n221 = Index Array(array=w357) -> (element=w360:cluster{string[]})  [unwired: 1 in]
            n222 = Unbundle(w356) -> ("Frame Rate"=w355:i32, "Compression"=w354:i32, "Size"=w358:u16)
            n223 = Unbundle(w360) -> (w359:string[])
            n224 = Index Array(array=w359, index=w358) -> (element=w353:string)
            n225 = call-poly <vilib>:"Write Key.vi"("section"=w364, "value"=w353, "key"="Size", "refnum"=w349) -> ("refnum out"=w366:T17)  [unwired: 2 in, 5 out]
            n226 = call-poly <vilib>:"Write Key.vi"("section"=w364, "value"=w355, "key"="FrameRate", "refnum"=w366) -> ("refnum out"=w365:T17)  [unwired: 1 in, 6 out]
            n227 = property on="Camera Settings" class="Clust (strict)"("Visible"=w367) -> ()  [unwired: 2 in, 2 out]
            n228 = local write "DB Camera Config"(w367) -> ()
            n229 = call-poly <vilib>:"Write Key.vi"("section"=w364, "value"=w354, "key"="Compression", "refnum"=w365) -> ("refnum out"=w351:T17)  [unwired: 1 in, 6 out]
            n230 = call <vilib>:"Close Config Data.vi"("refnum"=w351) -> ("file path"=w352:path)  [unwired: 2 in, 8 out]
            n231 = call <vilib>:"Open Config Data.vi"("configuration file path"=w352) -> ("refnum"=w350:T17)  [unwired: 8 in, 2 out]
          }
          frame True {
            n232 = property on="Camera Settings" class="Clust (strict)"("Visible"=TRUE) -> ()  [unwired: 2 in, 2 out]
          }
        }
      }
      event "Camera Settings": Value Change {
        n233 = event-data() -> ("NewVal"=w381:T2)  [unwired: 1 in]
        n234 = Index Array(array=w377) -> (element=w376:cluster{string[]})  [unwired: 1 in]
        n235 = Unbundle(w381) -> ("Frame Rate"=w372:i32, "Compression"=w371:i32, "Size"=w374:u16)
        n236 = Unbundle(w376) -> (w375:string[])
        n237 = Index Array(array=w375, index=w374) -> (element=w373:string)
        n238 = Format Into String(format string="%s   %dfps   %d%%", w373, w372, w371) -> (resulting string=w378:string)  [unwired: 2 in, 1 out]
        n239 = Build Array(w378) -> (w379:string[])
        n240 = property on="DB Camera Config" class="Bool (strict)"("Strings [4]"=w379) -> ()  [unwired: 2 in, 2 out]
      }
      event "Motor.Enable": Value Change {
        n241 = event-data() -> ("NewVal"=w387:bool)  [unwired: 1 in]
        n242 = Unbundle("Motor") -> ("Value"=w386:dbl)  [unwired: 1 out]
        n243 = Select(t=w386, s=w387, f=0.0) -> (s? t:f=w384:dbl)
        n244 = call <vilib>:"NT Write Number.vi"("Numeric"=w384, "Name"=w383) -> ()  [unwired: 9 in, 1 out]
      }
      event "Test Slider": Value Change {
        n245 = event-data() -> ("NewVal"=w390:dbl)  [unwired: 1 in]
        n246 = call <vilib>:"NT Write Number.vi"("Numeric"=w390, "Name"=w391) -> ()  [unwired: 9 in, 1 out]
      }
      event "On/Off": Value Change {
        n247 = event-data() -> ("NewVal"=w395:bool)  [unwired: 1 in]
        n248 = Boolean To (0,1)(Boolean=w395) -> (0, 1=w394:i16)
        n249 = call <vilib>:"NT Write Number.vi"("Numeric"=w394, "Name"=w393) -> ()  [unwired: 9 in, 1 out]
      }
      event "Rev/Fwd": Value Change {
        n250 = event-data() -> ("NewVal.Forward"=w403:bool, "NewVal.Reverse"=w402:bool)  [unwired: 1 in]
        n251 = Boolean To (0,1)(Boolean=w403) -> (0, 1=w399:i16)
        n252 = Boolean To (0,1)(Boolean=w402) -> (0, 1=w401:i16)
        n253 = Negate(x=w401) -> (-x=w400:i16)
        n254 = Add(x=w399, y=w400) -> (x+y=w398:i16)
        n255 = call <vilib>:"NT Write Number.vi"("Numeric"=w398, "Name"=w397) -> ()  [unwired: 9 in, 1 out]
      }
      event "Test Ring": Value Change {
        n256 = event-data() -> ("NewVal"=w407:u16)  [unwired: 1 in]
        n257 = property on="Test Ring" class="Ring (strict)"() -> ("Strings []"=w408:string[])  [unwired: 2 in, 2 out]
        n258 = Index Array(array=w408, index=w407) -> (element=w406:string)
        n259 = call <vilib>:"NT Write String.vi"("String"=w406, "Name"=w405) -> ()  [unwired: 9 in, 1 out]
      }
      event "Rec Mode": Value Change {
        # "Update globals for recording mode and path to read log from.\nClear when logging and let NetworkTables set path for vision to\nuse."
        n260 = event-data() -> ("NewVal"=w418:enum32{"Stop", "Record", "Playback"})  [unwired: 1 in]
        n261 = global write "WPI_DashboardLogging Global.vi" "Logging Filename"(path "") -> ()
        n262 = case shown="\"Stop\", \"Record\"" w418 {
          tunnel: w417 -> [_ w420 w428]
          tunnel: [_ _ w427] -> w414
          tunnel: [_ _ w426] -> _
          tunnel: w412 -> [_ _ w424]
          tunnel: cluster{i32, i32} {-250, 170} -> [_ _ w423]
          tunnel: [_ _ T19 {"Image Size"=TRUE, "Image Type"=TRUE, "Pixel Value"=TRUE, "ROI Information"=TRUE, "Zoom Factor"=FALSE} ("Image Information Shown:All Elements")] -> w410
          tunnel: [_ _ TRUE ("Zoom Factor")] -> w409
          frame Default {
          }
          frame "Stop", "Record" {
            # "Place Window too"
            n263 = invoke class="VI" method="FP.Close"(reference=w420) -> (reference out=w419:refnum<vi>)  [unwired: 2 in, 2 out]
            n264 = invoke class="VI" method="Abort VI"(reference=w419) -> ()  [unwired: 2 in, 3 out]
          }
          frame "Playback" {
            n265 = call "Open Playback Panel.vi"("Offset"=w423, "DB VI Ref"=w424, "Playback in"=w428) -> ("Playback out"=w425:refnum<vi>)  [unwired: 8 in]
            n266 = register-events(w425) -> (reference out=w427:refnum<event-registration>, error out=w426:errorcluster)  [unwired: 2 in]
          }
        }
        n267 = global write "WPI_DashboardLogging Global.vi" "Recording"(w418) -> ()
        n268 = property on="Camera Image" class="ImageControl"("Image Information Shown"=w410, "Image Information Visible"=w409) -> ()  [unwired: 2 in, 2 out]
        n269 = call <vilib>:"WPI_DashboardNT Log FieldName Cache.vi"("Operation"=enum16{"Lookup/Add", "Index", "Clear"}."Clear") -> ()  [unwired: 8 in, 3 out]
      }
      event Panel Close {
        w429 = enum32{"Stop", "Record", "Playback"}."Stop" ("Rec Mode")
        n270 = event-data() -> ()  [unwired: 1 in, 4 out]
        n271 = local write "Rec Mode"(w429) -> ()
        n272 = global write "WPI_DashboardLogging Global.vi" "Recording"(w429) -> ()
      }
      event Panel Close {
        # "Abort playback window and ourself"
        n273 = event-data() -> ()  [unwired: 1 in, 4 out]
        n274 = invoke class="VI" method="FP.Close"(reference=w434) -> (reference out=w433:refnum<vi>)  [unwired: 2 in, 2 out]
        n275 = invoke class="VI" method="Abort VI"(reference=w433) -> (error out=w432:errorcluster)  [unwired: 2 in, 2 out]
        n276 = invoke class="VI" method="Abort VI"(error in=w432) -> ()  [unwired: 2 in, 3 out]
      }
    }
  }
  n277 = property on="On/Off" class="Bool (strict)"("Visible"=w25) -> ()  [unwired: 2 in, 2 out]
  n278 = property on="Motor" class="Clust (strict)"("Visible"=w25) -> ()  [unwired: 2 in, 2 out]
  n279 = property on="Progress" class="Clust (strict)"("Visible"=w25) -> ()  [unwired: 2 in, 2 out]
  n280 = property on="Test Ring" class="Ring (strict)"("Visible"=w25) -> ()  [unwired: 2 in, 2 out]
  n281 = property on="Rev/Fwd" class="Clust (strict)"("Visible"=w25) -> ()  [unwired: 2 in, 2 out]
  n282 = property on="Camera Settings" class="Clust (strict)"("Visible"=w25) -> ()  [unwired: 2 in, 2 out]
  n283 = local write "DB Camera Config"(w25) -> ()
  n284 = global write "WPI_DashboardLogging Global.vi" "Recording"(w8) -> ()
  n285 = local write "Rec Mode"(w8) -> ()
